vi "Read Right Panel ref.vi"(8 "error in":errorcluster, 11 "Base Software in":refnum<class "Main.lvclass">) -> (0 "error out":errorcluster, 2 "Right Panel":refnum<vi>, 3 "Base Software out":refnum<class "Main.lvclass">)   [LabVIEW 2023, in "Main.lvlib" / "Main.lvclass"]
uses:
  Project/Main.lvclass
  Project/Main.lvclass/Main.ctl
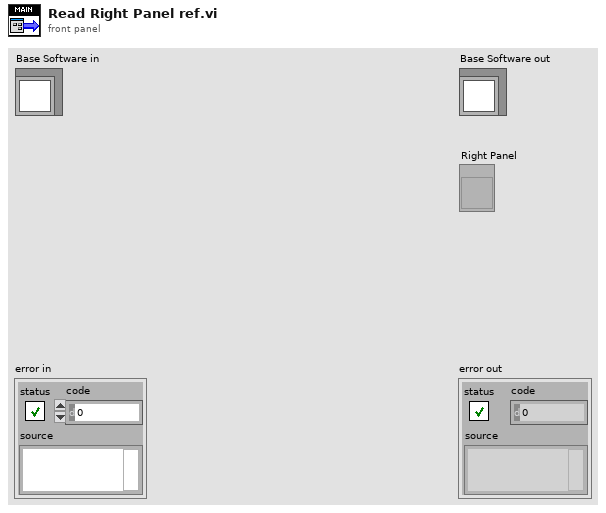
[diagram p1: front panel]
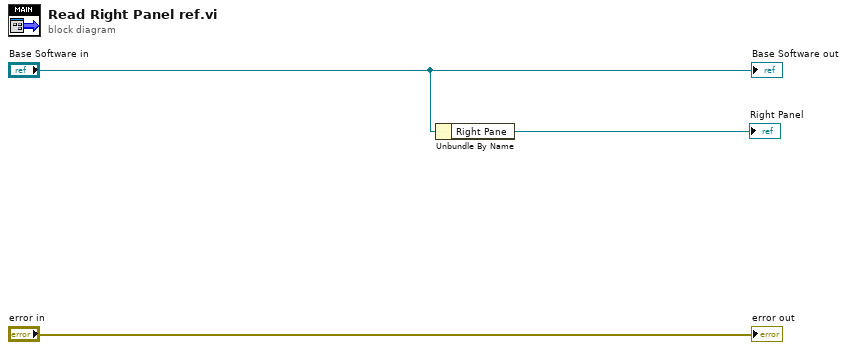
[diagram p0: block diagram]
diagram:
  n1 = Unbundle By Name("Base Software in") -> ("Right Pane"=→"Right Panel":refnum<vi>)
  "error out" <- "error in"
  "Base Software out" <- "Base Software in"
